vi "MT Measure PAM Quadrature Impairments.vi"(0 "recovered complex waveform":T6={"t0"=0.0, "dt"=1.0, "Y"=[]} {"Y" format="%.3f"; "dt" format="%^.2e"; "t0" format="%.4f"}, 1 "PAM system parameters":T3={"samples per symbol (16)"=16, "symbol map"=[]} {"symbol map" format="%.3f"}, 5 "input bit stream":i8[](array[numeric]), 7 "impairment measurement window":T4={"start index (symbols)"=0, "width (symbols) (-1: all)"=-1}, 11 "error in (no error)":errorcluster, 13 "reset? (T)":bool=TRUE) -> (2 "magnitude error":T1 {"individual symbol measurements (%)" format="%.2f"; "peak measurement (%)" format="%.2f"; "RMS measurement (%)" format="%.2f"}, 3 "DC offset measurements":T5 {"origin offset (dB)" format="%.2f"; "Q (%)" format="%.2f"; "I (%)" format="%.2f"}, 6 "phase error":T2 {"individual symbol measurements (deg)" format="%.2f"; "peak measurement (deg)" format="%.2f"; "RMS measurement (deg)" format="%.2f"}, 8 "EVM":T1 {"individual symbol measurements (%)" format="%.2f"; "peak measurement (%)" format="%.2f"; "RMS measurement (%)" format="%.2f"}, 10 "modulation error ratio (dB)":dbl format="%.2f", 15 "error out":errorcluster)   [LabVIEW 2020, in "niDMT.lvlib"]
doc: "This polymorphic instance calculates and reports pulse-amplitude modulation (PAM) quadrature impairments on a symbol-by-symbol basis at the symbol timing."
uses:
  <vilib>/addons/Modulation/niDMT.lvlib
  <vilib>/addons/Modulation/Analog/controls/Complex Data Waveform.ctl
  <vilib>/addons/Modulation/niAMT.lvlib
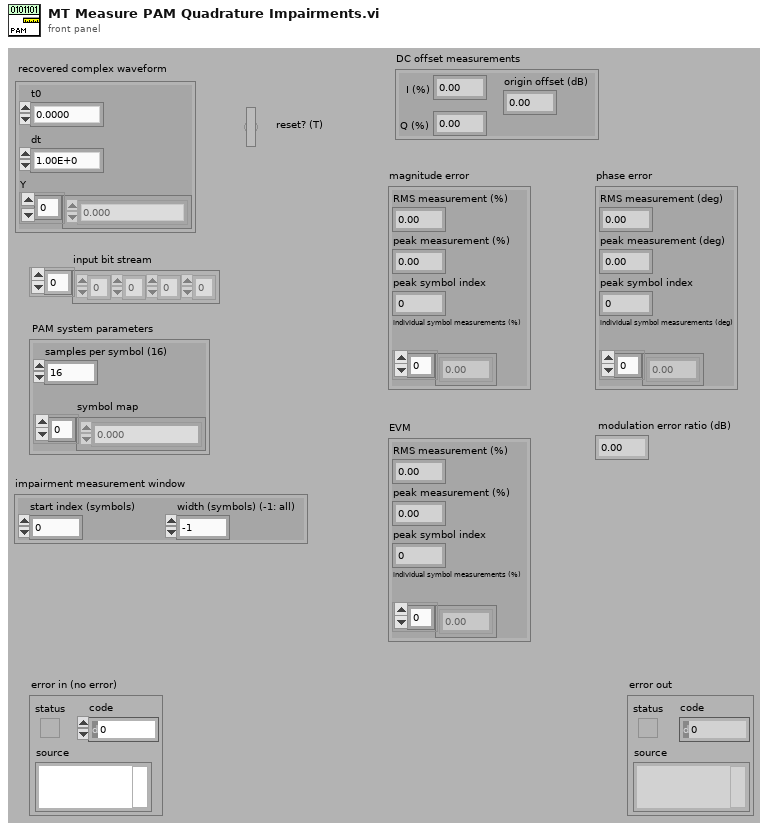
[diagram p1: front panel]
types:
  T1 = cluster{"RMS measurement (%)":dbl, "peak measurement (%)":dbl, "peak symbol index":i32, "individual symbol measurements (%)":dbl[]}
  T2 = cluster{"RMS measurement (deg)":dbl, "peak measurement (deg)":dbl, "peak symbol index":i32, "individual symbol measurements (deg)":dbl[]}
  T3 = cluster{"samples per symbol (16)":i32, "symbol map":cdb[]}
  T4 = cluster{"start index (symbols)":i32, "width (symbols) (-1: all)":i32}
  T5 = cluster{"I (%)":dbl, "Q (%)":dbl, "origin offset (dB)":dbl}
  T6 = typedef "niAMT.lvlib/Complex Data Waveform.ctl" = cluster{"t0":dbl, "dt":dbl, "Y":cdb[]}
  T7 = cluster{"I, %":dbl, "Q, %":dbl, "Origin Offset, dB":dbl}
  T8 = enum16{"FSK", "PSK", "QAM", "MSK", "PAM", "ASK", "CPM"}
  T9 = cluster{"RMS Measurement, %":dbl, "Peak Measurement, %":dbl, "Peak Symbol Index":i32, "Individual Symbol Measurements, %":dbl[]}
  T10 = cluster{"RMS Measurement, deg":dbl, "Peak Measurement, deg":dbl, "Peak Symbol Index":i32, "Individual Symbol Measurements, deg":dbl[]}
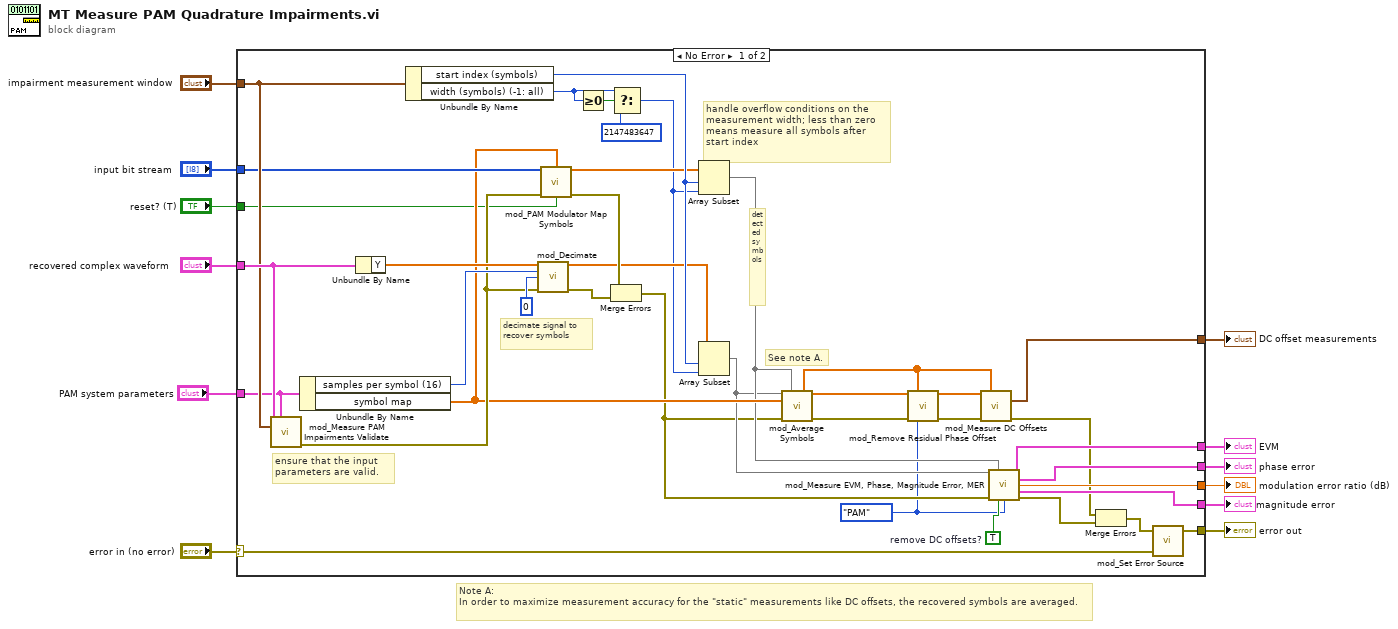
[diagram p0: block diagram]
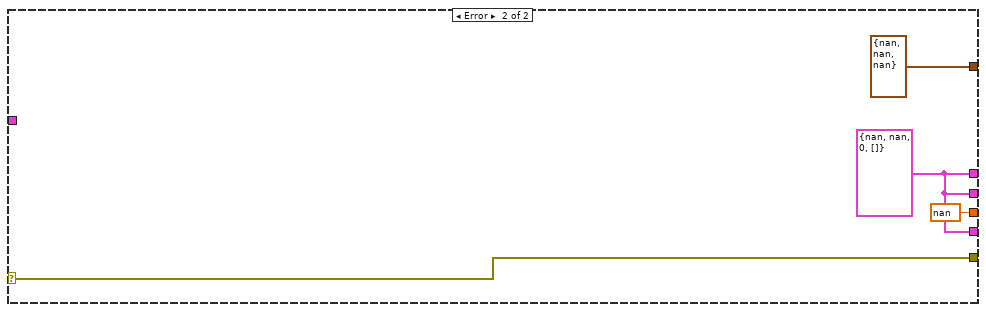
[diagram p2: hidden frame]
diagram:
  # "Note A:\nIn order to maximize measurement accuracy for the \"static\" measurements like DC offsets, the recovered symbols are averaged."
  n1 = case shown="No Error" "error in (no error)" {
    selector: "error in (no error)" -> [w42 w55]
    tunnel: "recovered complex waveform" -> [w49 _]
    tunnel: [w44 T7 {"I, %"=nan, "Q, %"=nan, "Origin Offset, dB"=nan} ("DC Offset Measurements")] -> w6
    tunnel: [w46 w53] -> w4
    tunnel: [w51 w53] -> w5
    tunnel: [w41 w55] -> w11
    tunnel: "input bit stream" -> [w36 _]
    tunnel: "impairment measurement window" -> [w47 _]
    tunnel: [w45 nan ("Modulation Error Ratio, dB")] -> w3
    tunnel: "PAM system parameters" -> [w39 _]
    tunnel: "reset? (T)" -> [w22 _]
    tunnel: [w17 w53] -> w1
    frame No Error {
      w13 = T8."PAM" ("Modulation Type")
      w23 = TRUE  # remove DC offsets?
      # "decimate signal to recover symbols"
      # "See note A."
      # "ensure that the input parameters are valid."
      # "detected symbols"
      # "handle overflow conditions on the\nmeasurement width; less than zero\nmeans measure all symbols after\nstart index"
      n2 = call <vilib>:"mod_Measure PAM Impairments Validate.vi"("Input Complex Waveform"=w49, "PAM System Parameters"=w39, "Impairment Measurement Window"=w47) -> ("error out"=w34:errorcluster)  [unwired: 12 out]
      n3 = Unbundle By Name(w39) -> ("samples per symbol (16)"=w38:i32, "symbol map"=w25:cdb[])
      n4 = Unbundle By Name(w49) -> ("Y"=w40:cdb[])
      n5 = Unbundle By Name(w47) -> ("start index (symbols)"=w48:i32, "width (symbols) (-1: all)"=w18:i32)
      n6 = call <vilib>:"mod_Decimate.vi"("Signal In"=w40, "Samples Per Symbol (16)"=w38, "Offset"=0, "error in (no error)"=w34) -> ("Signal Out"=w32:cdb[], "error out"=w31:errorcluster)  [unwired: 1 in, 9 out]
      n7 = call <vilib>:"mod_PAM Modulator Map Symbols.vi"("Input Bit Stream"=w36, "Symbol Map"=w25, "error in (no error)"=w34, "Reset? (T)"=w22) -> ("Symbols"=w35:cdb[], "error out"=w33:errorcluster)  [unwired: 10 out]
      n8 = Greater Or Equal To 0?(x=w18) -> (x >= 0?=w21:bool)
      n9 = Merge Errors(w33, w31) -> (w14:errorcluster)
      n10 = Select(t=w18, s=w21, f=2147483647) -> (s? t:f=w19:i32)
      n11 = Array Subset(array=w35, index=w48, length=w19) -> (w24:cdb[])
      n12 = Array Subset(array=w32, index=w48, length=w19) -> (w15:cdb[])
      n13 = call <vilib>:"mod_Average Symbols.vi"("Recovered Symbols"=w15, "Detected Symbols"=w24, "Symbol Map"=w25, "error in (no error)"=w14) -> ("Grouped Detected Symbols"=w28:cdb[], "Averaged Symbols"=w27:cdb[], "error out"=w30:errorcluster)  [unwired: 9 out]
      n14 = call <vilib>:"mod_Remove Residual Phase Offset.vi"("Averaged Symbols In"=w27, "Grouped Detected Symbols"=w28, "error in (no error)"=w30, "Modulation Type"=w13) -> ("Averaged Symbols Out"=w26:cdb[], "error out"=w29:errorcluster)  [unwired: 10 out]
      n15 = call <vilib>:"mod_Measure DC Offsets.vi"("Averaged Symbols"=w26, "Grouped Detected Symbols"=w28, "error in (no error)"=w29) -> ("DC Offset Measurements"=w44:T7, "error out"=w16:errorcluster)  [unwired: 1 in, 10 out]
      n16 = call <vilib>:"mod_Measure EVM, Phase, Magnitude Error, MER.vi"("Recovered Signal"=w15, "Detected Signal"=w24, "error in (no error)"=w14, "remove DC offsets? (T)"=w23, "Modulation Type"=w13) -> ("EVM"=w51:T9, "Phase Error"=w46:T10, "Modulation Error Ratio, dB"=w45:dbl, "magnitude error"=w17:T9, "error out"=w50:errorcluster)  [unwired: 1 in, 5 out]
      n17 = Merge Errors(w16, w50) -> (w43:errorcluster)
      n18 = call <vilib>:"mod_Set Error Source.vi"("initial error in (no error)"=w42, "final error in (no error)"=w43) -> ("error out"=w41:errorcluster)  [unwired: 3 out]
    }
    frame Error {
      w53 = T9 {"RMS Measurement, %"=nan, "Peak Measurement, %"=nan, "Peak Symbol Index"=0, "Individual Symbol Measurements, %"=[]} ("EVM")
    }
  }
  "error out" <- w11
  "modulation error ratio (dB)" <- w3
  "DC offset measurements" <- w6
  "EVM" <- w5
  "phase error" <- w4
  "magnitude error" <- w1
